vi "ADS1015 Config Formatter.vi"(11 "ADS1015 Config Options":T1={"I2C"={"Slave Address"=72, "Channel"=1}, "ADC"={"Channel"=0, "Expected Range (Programmable Gain Amplifier)"=0, "Sampling Mode"=0, "Sampling Rate"=0, "Comparator Mode"=0, "Comparator Polarity"=0, "Latching Comparator"=0, "Comparator Queue & Disable"=0}} {"ADC"."Comparator Queue & Disable" items=["Assert after one conversion", "Assert after two conversions", "Assert after four conversions", "Comparator disabled"]; "ADC"."Latching Comparator" items=["Non-latching", "Latching"]; "ADC"."Comparator Polarity" items=["Active Low", "Active High"]; "ADC"."Comparator Mode" items=["Traditional Comparator w/ hysteresis", "Window Comparator"]; "ADC"."Sampling Rate" items=["128SPS", "250SPS", "490SPS", "920SPS", "1600SPS", "2400SPS", "3300SPS"]; "ADC"."Sampling Mode" items=["Continuous Conversion", "Single-shot (Low Power)"]; "ADC"."Expected Range (Programmable Gain Amplifier)" items=["+/-6.144V", "+/-4.096V", "+/-2.048V", "+/-1.024V", "+/-0.512V", "+/-0.256V"]; "ADC"."Channel" items=["Differential: Ch 0&1", "Differential: Ch 0&3", "Differential: Ch 1&3", "Differential: Ch 2&3", "Single Ended: Ch 0", "Single Ended: Ch 1", "Single Ended: Ch 2", "Single Ended: Ch 3"]; "I2C"."Slave Address" format="%.0x"}) -> (3 "Config Command":u16=4096 format="%.0x")   [LabVIEW 2017]
uses:
  ADS1015 Config Options.ctl
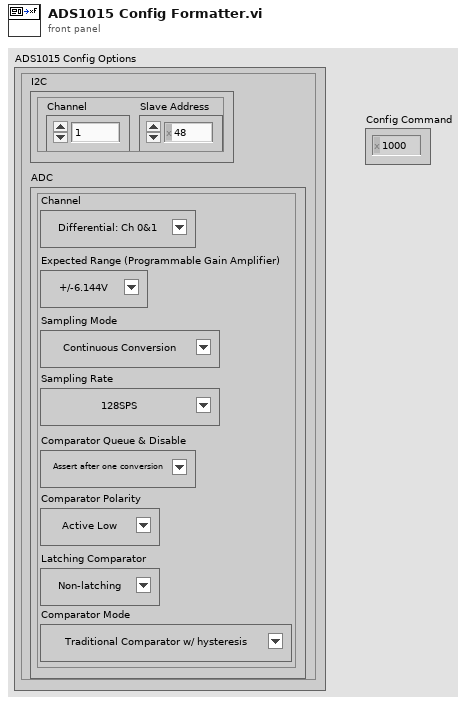
[diagram p1: front panel]
types:
  T1 = typedef "ADS1015 Config Options.ctl" = cluster{"I2C":cluster{"Slave Address":u8, "Channel":u8}, "ADC":cluster{"Channel":u8, "Expected Range (Programmable Gain Amplifier)":u8, "Sampling Mode":u8, "Sampling Rate":u8, "Comparator Mode":u8, "Comparator Polarity":u8, "Latching Comparator":u8, "Comparator Queue & Disable":u8}}
  T2 = cluster{"Channel":u8, "Expected Range (Programmable Gain Amplifier)":u8, "Sampling Mode":u8, "Sampling Rate":u8, "Comparator Mode":u8, "Comparator Polarity":u8, "Latching Comparator":u8, "Comparator Queue & Disable":u8}
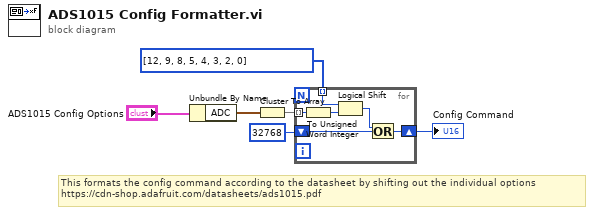
[diagram p0: block diagram]
diagram:
  # "This formats the config command according to the datasheet by shifting out the individual options\nhttps://cdn-shop.adafruit.com/datasheets/ads1015.pdf"
  n1 = Unbundle By Name("ADS1015 Config Options") -> ("ADC"=w1:T2)
  n2 = Cluster To Array(cluster=w1) -> (array=w6:u8[])
  n3 = for {
    tunnel: w6 -> [w12] mode=indexing
    tunnel: i16[] [12, 9, 8, 5, 4, 3, 2, 0] -> [w11] mode=indexing
    shift-right: [w9] -> w3
    shift-left: u16 32768 -> [w8]
    n4 = To Unsigned Word Integer(number=w12) -> (unsigned 16bit integer=w7:u16)
    n5 = Logical Shift(y=w11, x=w7) -> (x << y=w10:u16)
    n6 = Or(x=w10, y=w8) -> (x .or. y?=w9:u16)
  }
  "Config Command" <- w3
